vi "GetConnectedPumps.vi"(0 "object in":refnum<class "CetoniPump.lvclass">, 5 "error in (no error)":errorcluster) -> (14 "object out":refnum<class "CetoniPump.lvclass">, 15 "ConnectedPumps":T1(array[cluster]), 19 "error out":errorcluster)   [LabVIEW 2021, in "CetoniPump.lvclass"]
uses:
  CetoniPump.lvclass
  CetoniPump.lvclass/CetoniPump.ctl
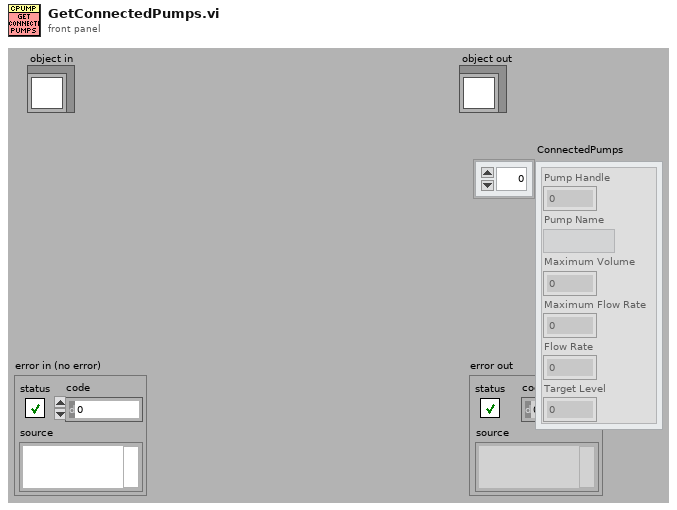
[diagram p1: front panel]
types:
  T1 = cluster{"Pump Handle":i64, "Pump Name":string, "Maximum Volume":dbl, "Maximum Flow Rate":dbl, "Flow Rate":dbl, "Target Level":dbl}[]
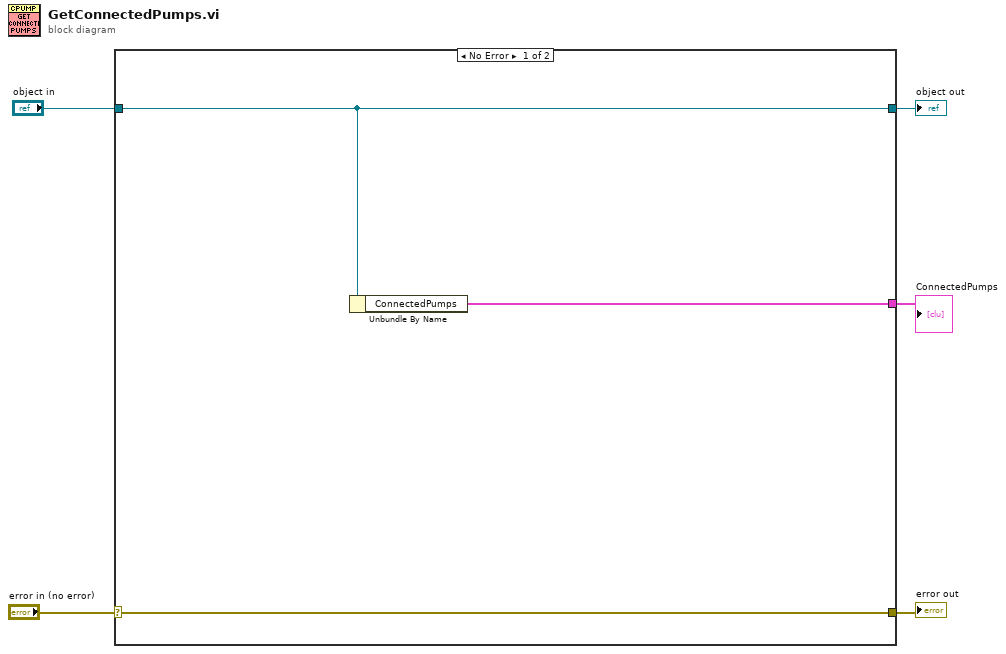
[diagram p0: block diagram]
diagram:
  n1 = case shown="No Error" "error in (no error)" {
    selector: "error in (no error)" -> [w7 w10]
    tunnel: [w7 w10] -> w4
    tunnel: [w6 w9] -> w2
    tunnel: "object in" -> [w6 w9]
    tunnel: [w8 _] -> w1
    frame No Error {
      n2 = Unbundle By Name(w6) -> ("ConnectedPumps"=w8:T1)
    }
    frame Error {
    }
  }
  "error out" <- w4
  "object out" <- w2
  "ConnectedPumps" <- w1
